vi "ArrayBreakup.vi"(8 "error in (no error)":errorcluster caption="错误输入", 11 "ArrayIn":string[](array[string])=["123", "345", "456", "789", "901"]) -> (0 "error out":errorcluster caption="错误输出", 2 "Array2":string[](array[string]), 3 "Array1":string[](array[string]))   [LabVIEW 2013]
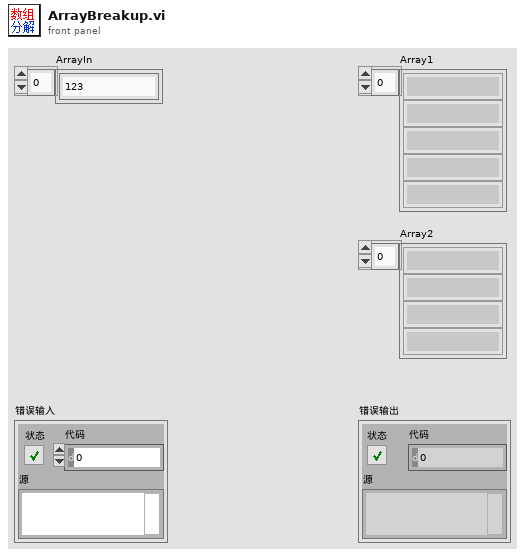
[diagram p1: front panel]
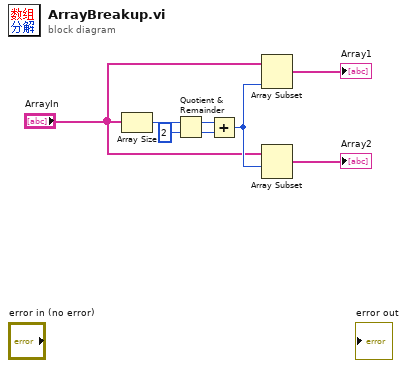
[diagram p0: block diagram]
diagram:
  n1 = Array Size(array="ArrayIn") -> (size(s)=w8:i32)
  n2 = Quotient & Remainder(x=w8, y=2) -> (x-y*floor(x/y)=w5:i32, floor(x/y)=w6:i32)
  n3 = Add(x=w5, y=w6) -> (x+y=w4:i32)
  n4 = Array Subset(array="ArrayIn", length=w4) -> (→"Array1":string[])  [unwired: 1 in]
  n5 = Array Subset(array="ArrayIn", index=w4) -> (→"Array2":string[])  [unwired: 1 in]
